vi "Cluster_Get Element Data for Tree.vi"(10 "Nest Chain":string[](array[string]), 11 "Data Type":variant) -> (3 "Cluster Element Data Aray":T1[](array[typedef]))   [LabVIEW 2023]
uses:
  Cluster Element Description.ctl
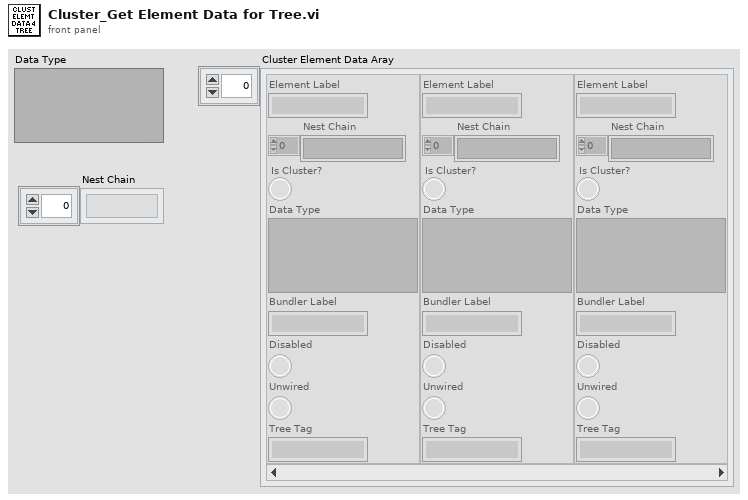
[diagram p1: front panel]
types:
  T1 = typedef "Cluster Element Description.ctl" = cluster{"Element Label":string, "Nest Chain":string[], "Is Cluster?":bool, "Data Type":variant, "Bundler Label":string, "Disabled":bool, "Unwired":bool, "Tree Tag":string}
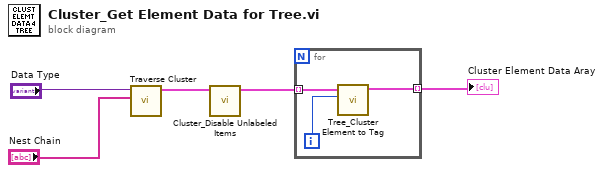
[diagram p0: block diagram]
diagram:
  n1 = call "Traverse Cluster.vi"("Nest Chain"="Nest Chain", "Data Type"="Data Type") -> ("Array"=w2:T1[])  [unwired: 9 in]
  n2 = call "Cluster_Disable Unlabeled Items.vi"("Cluster Items"=w2) -> ("Cluster Items Out"=w1:T1[])  [unwired: 10 in]
  n3 = for {
    tunnel: w1 -> [w8] mode=indexing
    tunnel: [w6] -> w3 mode=indexing
    i -> [w7]
    n4 = call "Tree_Cluster Element to Tag.vi"("Index"=w7, "Cluster Element Data"=w8) -> ("Cluster Element Data Out"=w6:T1)  [unwired: 8 in, 1 out]
  }
  "Cluster Element Data Aray" <- w3
